vi "Forward BP Trigger.vi"(0 "fpga reference in":refnum<k20>[](array[refnum]), 5 "Board Settings in":T1[](array[typedef]) {"Address Space" items=["VXI/VME A16"=1, "VXI/VME A24"=2, "VXI/VME A32"=3, "VXI/VME A64"=4, "PXI Memory Allocations"=9, "PXI Configuration"=10, "PXI BAR0"=11, "PXI BAR1"=12, "PXI BAR2"=13, "PXI BAR3"=14, "PXI BAR4"=15, "PXI BAR5"=16]}, 11 "error in":errorcluster) -> (4 "fpga reference out":refnum<k20>[](array[refnum]), 6 "Board Settings out":T1[](array[typedef]) {"Address Space" items=["VXI/VME A16"=1, "VXI/VME A24"=2, "VXI/VME A32"=3, "VXI/VME A64"=4, "PXI Memory Allocations"=9, "PXI Configuration"=10, "PXI BAR0"=11, "PXI BAR1"=12, "PXI BAR2"=13, "PXI BAR3"=14, "PXI BAR4"=15, "PXI BAR5"=16]}, 15 "error out":errorcluster)   [LabVIEW 2019]
uses:
  <instrlib>/niMmWave/ni3610 and ni3630/controls/public/Main Settings.ctl
  <vilib>/Instr/_visa.llb/VISA Register Access Address Space.ctl
  <instrlib>/niMmWave/ni3610 and ni3630/controls/public/Register Adresses.ctl
  <instrlib>/niMmWave/ni3610 and ni3630/controls/public/Base Card Type.ctl
  <instrlib>/niMmWave/ni3610 and ni3630/controls/private/IQ Card Revision.ctl
  <instrlib>/niMmWave/ni3610 and ni3630/controls/public/Board Capability.ctl
  <instrlib>/niMmWave/ni3610 and ni3630/controls/public/SPI Cmd.ctl
  <instrlib>/niMmWave/ni3610 and ni3630/controls/public/Trigger Source.ctl
  <instrlib>/niMmWave/ni3610 and ni3630/controls/public/Trigger Sink.ctl
  TypeDefs/Shared FPGA Reference.ctl
  <vilib>/Utility/error.llb/Error Cluster From Error Code.vi
  <vilib>/rvi/errors/niLvFpgaAdjustHostInterfaceError.vi
  <vilib>/rvi/interface/nirviReadWriteControl/nirviReadWriteControl.xnode
  <instrlib>/niMmWave/ni3610 and ni3630/ni3610_and_ni3630_Driver_Lib.lvlib
  NiFpgaLv.dll
  <vilib>/rvi/interface/Simulation/niFpgaSimulationCallBeginRW.vi
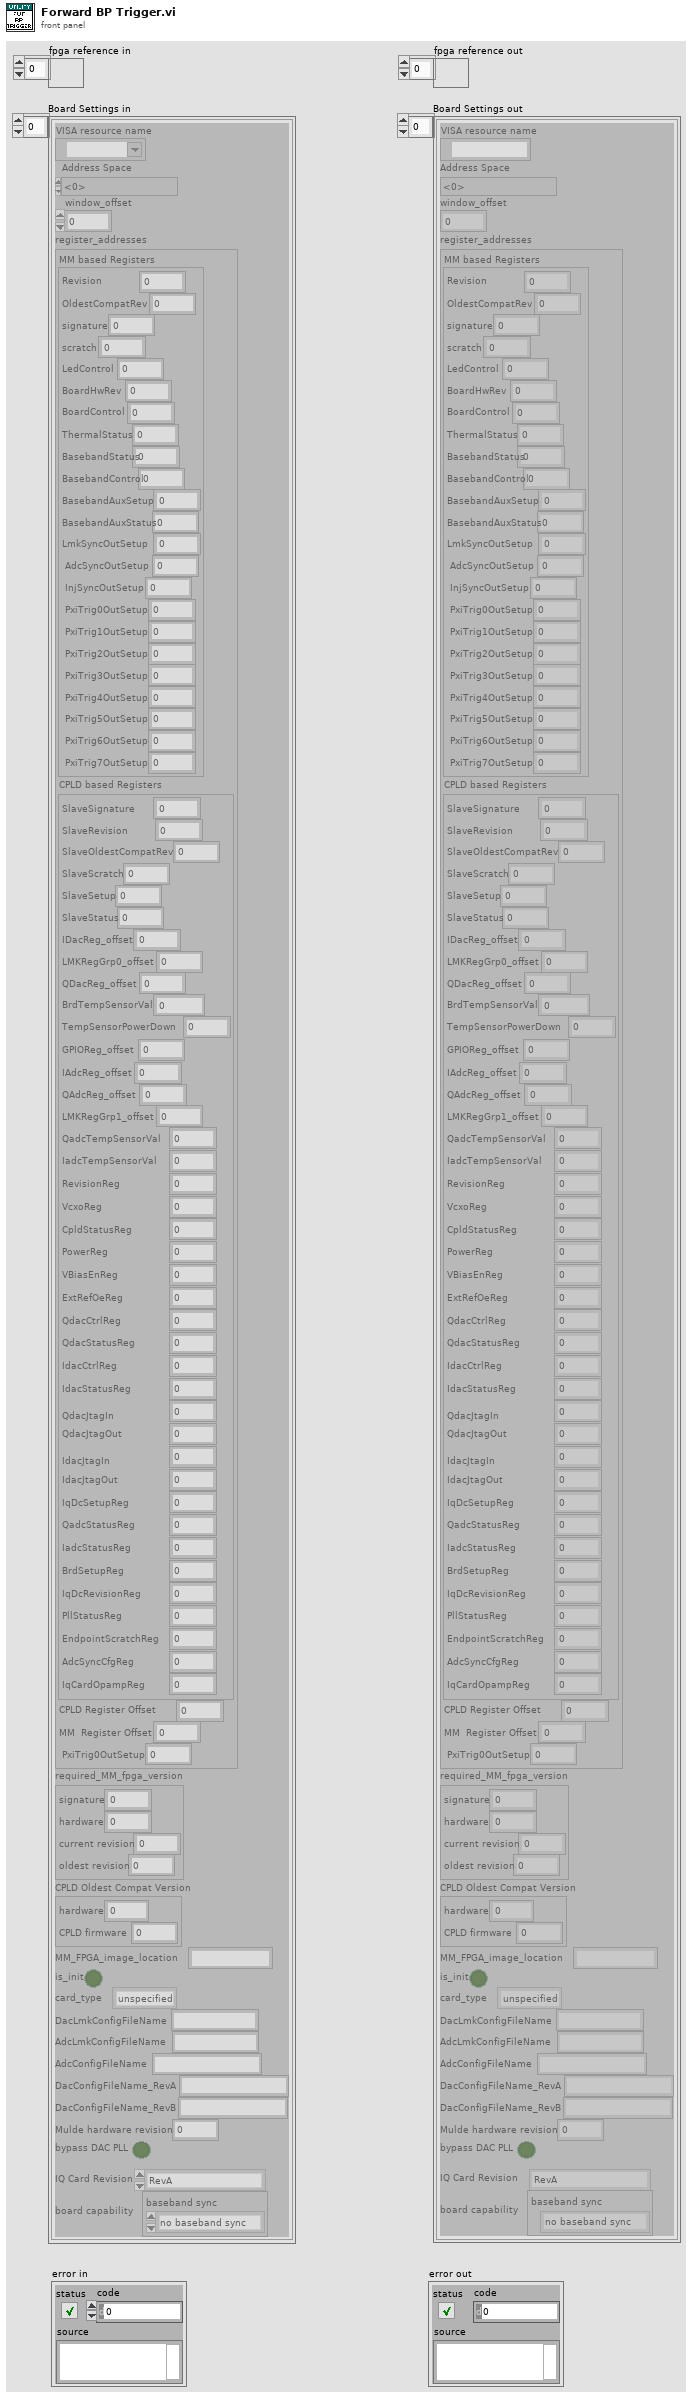
[diagram p1: front panel]
types:
  T1 = typedef "ni3610_and_ni3630_Driver_Lib.lvlib/Main Settings.ctl" = cluster{"VISA resource name":refnum<visa-resource-name>, "Address Space":T2, "window_offset":u32, "register_addresses":T3, "required_MM_fpga_version":cluster{"signature":u32, "hardware":u32, "current revision":u32, "oldest revision":u32}, "CPLD Oldest Compat Version ":cluster{"hardware":u32, "CPLD firmware":u32}, "MM_FPGA_image_location":string, "is_init":bool, "card_type":T4, "DacLmkConfigFileName":string, "AdcLmkConfigFileName":string, "AdcConfigFileName":string, "DacConfigFileName_RevA":string, "DacConfigFileName_RevB":string, "Mulde hardware revision":u8, "bypass DAC PLL\n":bool, "IQ Card Revision":T5, "board capability":T6}
  T2 = typedef "VISA Register Access Address Space.ctl" = u16
  T3 = typedef "ni3610_and_ni3630_Driver_Lib.lvlib/Register Adresses.ctl" = cluster{"MM based Registers":cluster{"Revision":u32, "OldestCompatRev":u32, "signature":u32, "scratch":u32, "LedControl":u32, "BoardHwRev":u32, "BoardControl":u32, "ThermalStatus":u32, "BasebandStatus":u32, "BasebandControl":u32, "BasebandAuxSetup":u32, "BasebandAuxStatus":u32, "LmkSyncOutSetup":u32, " AdcSyncOutSetup":u32, " InjSyncOutSetup":u32, " PxiTrig0OutSetup":u32, " PxiTrig1OutSetup":u32, " PxiTrig2OutSetup":u32, " PxiTrig3OutSetup":u32, " PxiTrig4OutSetup":u32, " PxiTrig5OutSetup":u32, " PxiTrig6OutSetup":u32, " PxiTrig7OutSetup":u32}, "CPLD based Registers":cluster{"SlaveSignature":u32, "SlaveRevision":u32, "SlaveOldestCompatRev":u32, "SlaveScratch":u32, "SlaveSetup":u32, "SlaveStatus":u32, "IDacReg_offset":u32, "LMKRegGrp0_offset":u32, "QDacReg_offset":u32, "BrdTempSensorVal":u32, "TempSensorPowerDown":u32, "GPIOReg_offset":u32, "IAdcReg_offset":u32, "QAdcReg_offset":u32, "LMKRegGrp1_offset":u32, "QadcTempSensorVal":u32, "IadcTempSensorVal":u32, "RevisionReg":u32, "VcxoReg":u32, "CpldStatusReg":u32, "PowerReg":u32, "VBiasEnReg":u32, "ExtRefOeReg":u32, "QdacCtrlReg":u32, "QdacStatusReg":u32, "IdacCtrlReg":u32, "IdacStatusReg":u32, "QdacJtagIn":u32, "QdacJtagOut":u32, "IdacJtagIn":u32, "IdacJtagOut":u32, "IqDcSetupReg":u32, "QadcStatusReg":u32, "IadcStatusReg":u32, "BrdSetupReg":u32, "IqDcRevisionReg":u32, "PllStatusReg":u32, "EndpointScratchReg":u32, "AdcSyncCfgReg":u32, "IqCardOpampReg":u32}, "CPLD Register Offset":u32, "MM  Register Offset":u32, " PxiTrig0OutSetup":u32}
  T4 = typedef "ni3610_and_ni3630_Driver_Lib.lvlib/Base Card Type.ctl" = enum16{"unspecified", "ADC", "DAC"}
  T5 = typedef "ni3610_and_ni3630_Driver_Lib.lvlib/IQ Card Revision.ctl" = enum16{"RevA", "RevB", "RevC", "RevD"}
  T6 = typedef "ni3610_and_ni3630_Driver_Lib.lvlib/Board Capability.ctl" = cluster{"baseband sync":enum16{"no baseband sync", "baseband sync"}}
  T7 = typedef "ni3610_and_ni3630_Driver_Lib.lvlib/Trigger Source.ctl" = enum16{"CntrlDisabled", "LmkSysRef ", "LmkDevClk", "OrDacSync ", "AndDacSync ", "IDacSync", "QDacSync "}
  T8 = typedef "ni3610_and_ni3630_Driver_Lib.lvlib/Trigger Sink.ctl" = enum16{"LmkSyncOutSetup", "AdcSyncOutSetup", "InjSyncOutSetup"}
  T9 = typedef "ni3610_and_ni3630_Driver_Lib.lvlib/SPI Cmd.ctl" = cluster{"SPI address":u32, "SPI data":u32}
  T10 = typedef "Shared FPGA Reference.ctl" = refnum<k20>
  T11 = cluster{"control":cluster{"measure tdc":bool, "enable measurement":bool, "10 kHz tclk enable":bool, "200 kHz tclk enable":bool, "output enable":bool, "reset":bool, "deassert holdoff":u8, "calibrate":bool, "calibrate width":u8, "tclk trigger enable":bool, "alignment complete":bool}, "tclk parameters":cluster{"rollover count":u16, "rising edge count":u16, "falling edge count":u16}}
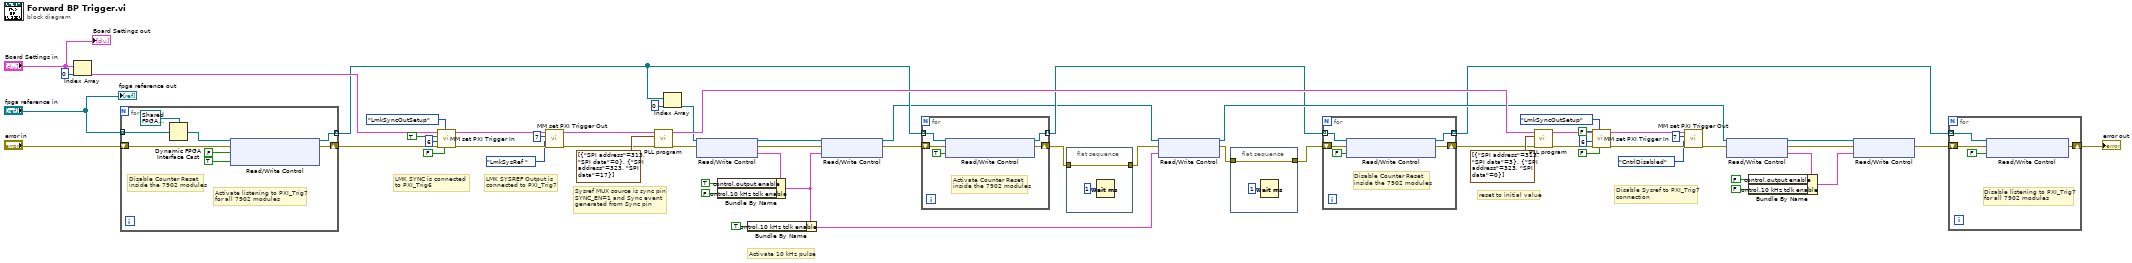
[diagram p0: block diagram]
diagram:
  # "Disable Sysref to PXI_Trig7\nconnection"
  # "reset to initial value"
  # "Activate 10 kHz pulse"
  # "LMK SYSREF Output is \nconnected to PXI_Trig7"
  # "LMK SYNC is connected\nto PXI_Trig6"
  # "Sysref MUX source is sync pin\nSYNC_EN=1 and Sync event\ngenerated from Sync pin"
  n1 = Index Array(array="Board Settings in", index=0) -> (element=w36:T1)
  n2 = for {
    shift-right: [w65] -> w39
    shift-left: "error in" -> [w62]
    tunnel: [w66] -> w7 mode=indexing
    tunnel: "fpga reference in" -> [w68] mode=indexing
    # "Disable Counter Reset\ninside the 7902 modules"
    # "Activate listening to PXI_Trig7\nfor all 7902 modules"
    n3 = Dynamic FPGA Interface Cast(Session In=T10 refnum ("fpga reference"), Type=w68) -> (Session Out=w61:T10)
    n4 = xnode "Read/Write Control"("FPGA VI Reference In"=w61, "error in"=w62, "sync.counter reset enable"=FALSE ("Master Reset Enable"), "sync.master reset listen"=TRUE ("master reset listen")) -> ("FPGA VI Reference Out"=w66:T10, "error out"=w65:errorcluster)
  }
  n5 = call <instrlib>:"MM set PXI Trigger In.vi"("Force Enable"=FALSE, "Trigger Sink"=Trigger_Sink."LmkSyncOutSetup", "error in"=w39, "PXI Trigger Select (0..7)"=u8 6, "Enable Trigger Input"=TRUE, "Board Settings in"=w36) -> ("error out"=w44:errorcluster, "Board Settings out"=w45:T1)  [unwired: 4 in]
  n6 = call <instrlib>:"MM set PXI Trigger Out.vi"("error in"=w44, "Trigger Source"=Trigger_Source."LmkSysRef ", "PXI Trigger Select (0..7)"=u8 7, "Board Settings in"=w45) -> ("error out"=w43:errorcluster, "Board Settings out"=w42:T1)  [unwired: 6 in]
  n7 = call <instrlib>:"PLL program.vi"("error in"=w43, "SPI settings array"=T9[] [{"SPI address"=313, "SPI data"=0}, {"SPI address"=323, "SPI data"=17}], "Board Settings in"=w42) -> ("error out"=w38:errorcluster, "Board Settings out"=w20:T1)  [unwired: 7 in]
  n8 = Index Array(array=w7, index=0) -> (element=w15:T10)
  n9 = xnode "Read/Write Control"("FPGA VI Reference In"=w15, "error in"=w38) -> ("FPGA VI Reference Out"=w5:T10, "error out"=w1:errorcluster, "sync.parameters"=w54:T11)
  n10 = Bundle By Name(cluster=w54, "control.output enable"=TRUE, "control.10 kHz tclk enable"=FALSE ("control.pulse injection")) -> (w50:T11)
  n11 = Bundle By Name(cluster=w50, "control.10 kHz tclk enable"=TRUE ("control.measure")) -> (w53:T11)
  n12 = xnode "Read/Write Control"("FPGA VI Reference In"=w5, "error in"=w1, "sync.parameters"=w50) -> ("FPGA VI Reference Out"=w2:T10, "error out"=w4:errorcluster)
  n13 = for {
    shift-right: [w72] -> w3
    shift-left: w4 -> [w73]
    tunnel: w7 -> [w70] mode=indexing
    tunnel: [w69] -> w6 mode=indexing
    # "Activate Counter Reset\ninside the 7902 modules"
    n14 = xnode "Read/Write Control"("FPGA VI Reference In"=w70, "error in"=w73, "sync.counter reset enable"=TRUE ("Master Reset Enable")) -> ("FPGA VI Reference Out"=w69:T10, "error out"=w72:errorcluster)
  }
  n15 = flat-sequence {
    tunnel: w3 -> [w74]
    tunnel: [w74] -> w52
    frame #0 {
      n16 = Wait (ms)(milliseconds to wait=u32 1) -> ()  [unwired: 1 out]
    }
  }
  n17 = xnode "Read/Write Control"("FPGA VI Reference In"=w2, "error in"=w52, "sync.parameters"=w53) -> ("FPGA VI Reference Out"=w9:T10, "error out"=w51:errorcluster)
  n18 = flat-sequence {
    tunnel: w51 -> [w76]
    tunnel: [w76] -> w11
    frame #0 {
      n19 = Wait (ms)(milliseconds to wait=u32 1) -> ()  [unwired: 1 out]
    }
  }
  n20 = for {
    shift-right: [w81] -> w10
    shift-left: w11 -> [w82]
    tunnel: w6 -> [w79] mode=indexing
    tunnel: [w78] -> w8 mode=indexing
    # "Disable Counter Reset\ninside the 7902 modules"
    n21 = xnode "Read/Write Control"("FPGA VI Reference In"=w79, "error in"=w82, "sync.counter reset enable"=FALSE ("Master Reset Enable")) -> ("FPGA VI Reference Out"=w78:T10, "error out"=w81:errorcluster)
  }
  n22 = call <instrlib>:"PLL program.vi"("error in"=w10, "SPI settings array"=T9[] [{"SPI address"=313, "SPI data"=3}, {"SPI address"=323, "SPI data"=0}], "Board Settings in"=w20) -> ("error out"=w26:errorcluster, "Board Settings out"=w27:T1)  [unwired: 7 in]
  n23 = call <instrlib>:"MM set PXI Trigger In.vi"("Force Enable"=FALSE, "Trigger Sink"=Trigger_Sink."LmkSyncOutSetup", "error in"=w26, "PXI Trigger Select (0..7)"=u8 6, "Enable Trigger Input"=FALSE, "Board Settings in"=w27) -> ("error out"=w32:errorcluster, "Board Settings out"=w31:T1)  [unwired: 4 in]
  n24 = call <instrlib>:"MM set PXI Trigger Out.vi"("error in"=w32, "Trigger Source"=Trigger_Source."CntrlDisabled", "PXI Trigger Select (0..7)"=u8 7, "Board Settings in"=w31) -> ("error out"=w21:errorcluster)  [unwired: 6 in, 1 out]
  n25 = xnode "Read/Write Control"("FPGA VI Reference In"=w9, "error in"=w21) -> ("FPGA VI Reference Out"=w58:T10, "error out"=w14:errorcluster, "sync.parameters"=w56:T11)
  n26 = Bundle By Name(cluster=w56, "control.output enable"=FALSE, "control.10 kHz tclk enable"=FALSE ("control.pulse injection")) -> (w55:T11)
  n27 = xnode "Read/Write Control"("FPGA VI Reference In"=w58, "error in"=w14, "sync.parameters"=w55) -> ("error out"=w13:errorcluster)  [unwired: 1 out]
  n28 = for {
    shift-right: [w86] -> w18
    shift-left: w13 -> [w84]
    tunnel: w8 -> [w83] mode=indexing
    # "Disable listening to PXI_Trig7\nfor all 7902 modules"
    n29 = xnode "Read/Write Control"("FPGA VI Reference In"=w83, "error in"=w84, "sync.master reset listen"=FALSE ("control.measure")) -> ("error out"=w86:errorcluster)  [unwired: 1 out]
  }
  "error out" <- w18
  "Board Settings out" <- "Board Settings in"
  "fpga reference out" <- "fpga reference in"
